vi "MeasureRMSJ&J.vi"(9 "#of Samples":dbl, 10 "Sampling Rate":dbl) -> (1 "(Vrms)":dbl format="%0.2f", 2 "Waveform Graph":dbl[](graph))   [LabVIEW 2015]
uses:
  <vilib>/Analysis/NI_AALPro.lvlib
panel:
  out "Numeric":i32
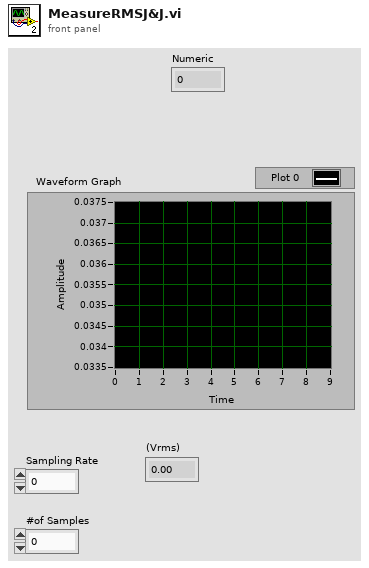
[diagram p1: front panel]
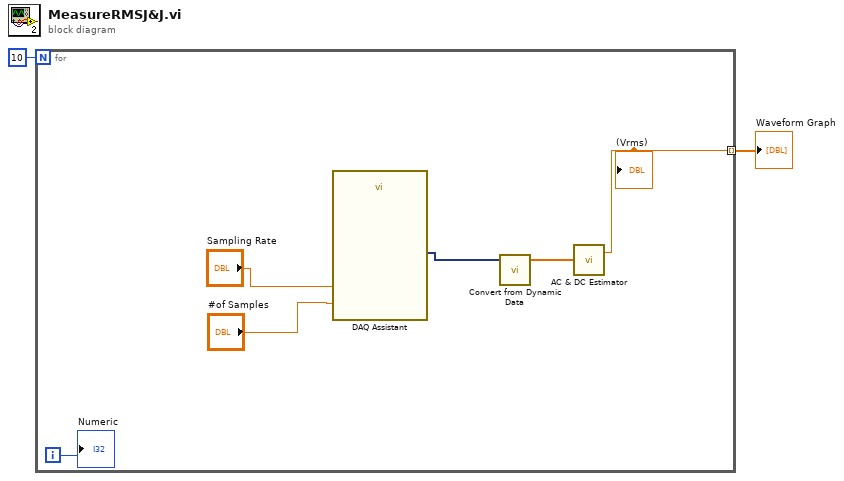
[diagram p0: block diagram]
diagram:
  n1 = for {
    N: 10 -> [_]
    tunnel: [w6] -> w2 mode=indexing
    i -> [w3]
    n2 = call "DAQ Assistant"("rate"="Sampling Rate", "number of samples"="#of Samples") -> ("data"=w8:dynamicdata)  [unwired: 15 in, 2 out]
    n3 = call "Convert from Dynamic Data"("Dynamic Data Type"=w8) -> ("Array"=w7:dbl[])  [unwired: 3 in]
    n4 = call <vilib>:"AC & DC Estimator.vi"("Signal (V)"=w7) -> ("AC estimate (Vrms)"=w6:dbl)  [unwired: 1 out]
    "(Vrms)" <- w6
    "Numeric" <- w3
  }
  "Waveform Graph" <- w2
